vi "RobotProfileParser.vi"(0 "Selected Robot":i32) -> ()   [LabVIEW 2019]
doc: "Uses robot profile information to determine which sensors should be bypassed"
uses:
  robotprofile.vi
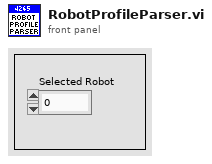
[diagram p1: front panel]
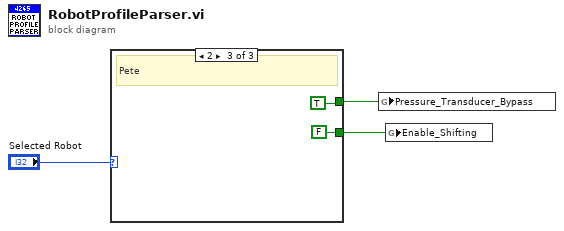
[diagram p0: block diagram]
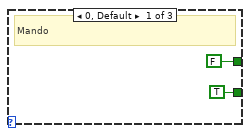
[diagram p2: hidden frame]
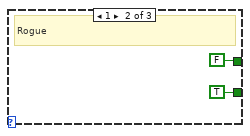
[diagram p3: hidden frame]
diagram:
  n1 = case shown="2" "Selected Robot" {
    tunnel: [FALSE ("Pressure_Transducer_Bypass") FALSE ("Pressure_Transducer_Bypass") TRUE ("Pressure_Transducer_Bypass")] -> w2
    tunnel: [TRUE ("Pressure_Transducer_Bypass") TRUE ("Pressure_Transducer_Bypass") FALSE ("Pressure_Transducer_Bypass")] -> w1
    frame 0, Default {
      # "Mando"
    }
    frame 1 {
      # "Rogue"
    }
    frame 2 {
      # "Pete"
    }
  }
  n2 = global write "robotprofile.vi" "Pressure_Transducer_Bypass"(w2) -> ()
  n3 = global write "robotprofile.vi" "Enable_Shifting"(w1) -> ()
